vi "AddActions.vi"(0 "object in":refnum<class "StateReverse.lvclass">, 1 "StatesIn":T1[](array[typedef]), 5 "error in (no error)":errorcluster, 6 "StateStrings":string[](array[string]), 8 "StateActions":cluster{"StateActions":string[]}[](array[cluster]), 10 "StateComments":cluster{"StateActions":string[]}[](array[cluster])) -> (14 "object out":refnum<class "StateReverse.lvclass">, 15 "States":T1[](array[typedef]), 19 "error out":errorcluster)   [LabVIEW 2014, in "StateReverse.lvclass"]
uses:
  <resource>/Framework/Providers/Open_GDS/UML/StateReverse_class/StateReverse.lvclass
  <resource>/Framework/Providers/Open_GDS/UML/ReversedEngineering/ReversedEngineering StateMachineStateInfo.ctl
  <resource>/Framework/Providers/Open_GDS/UML/StateReverse_class/StateReverse.lvclass/StateReverse.ctl
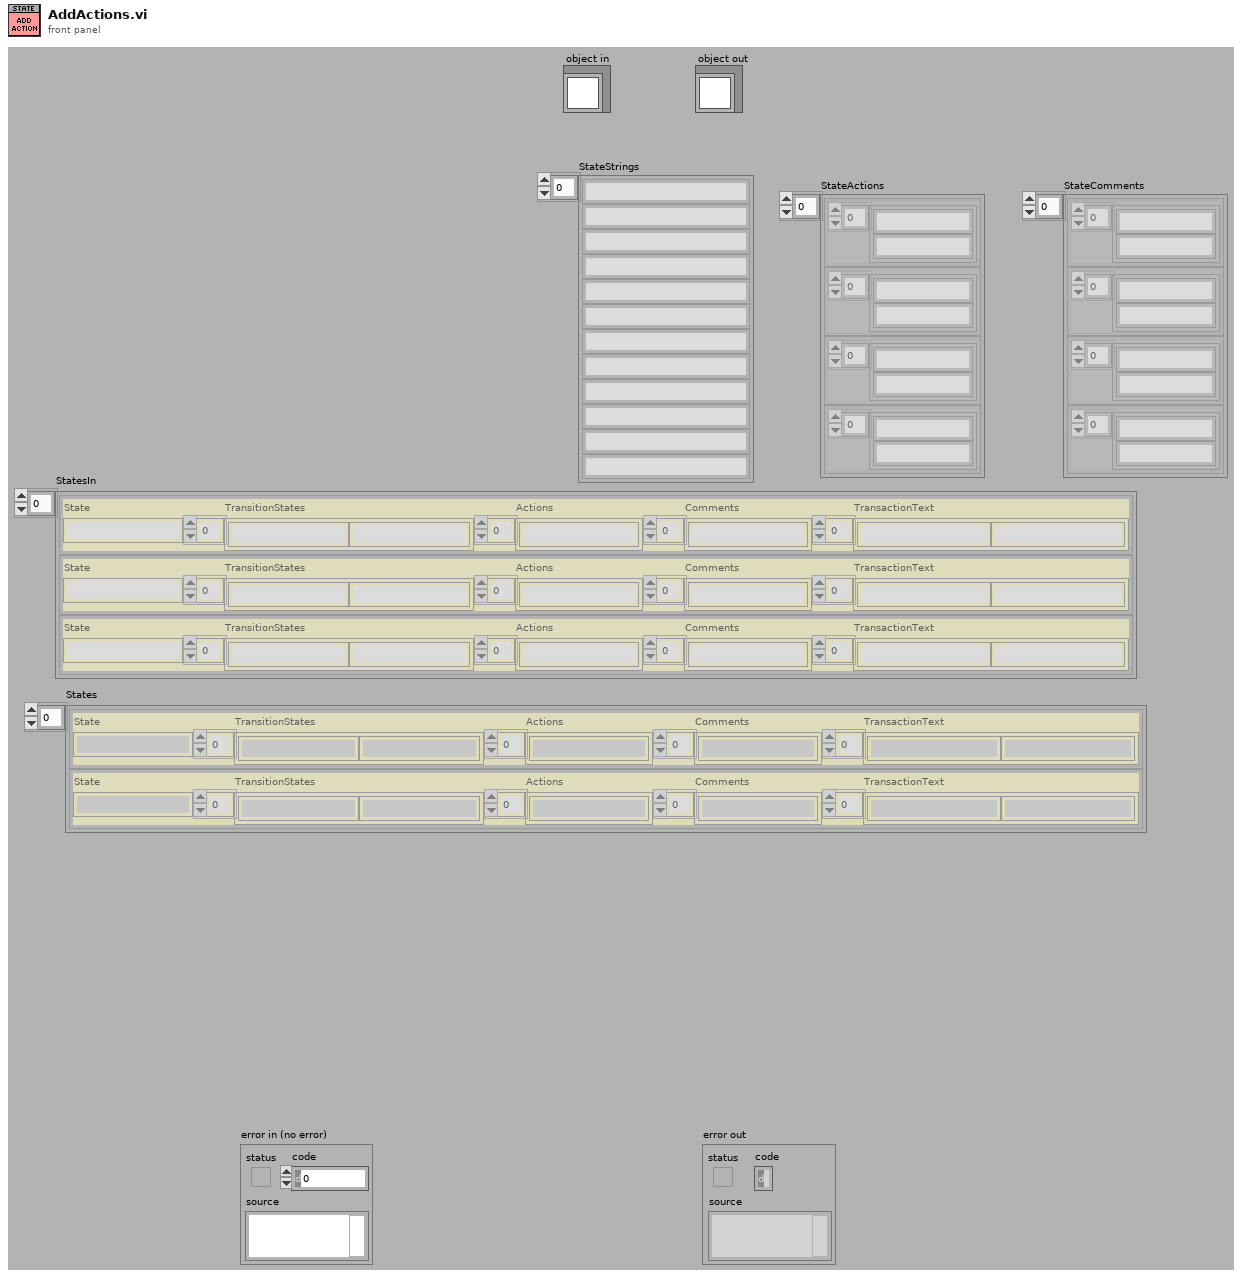
[diagram p1: front panel]
types:
  T1 = typedef "ReversedEngineering StateMachineStateInfo.ctl" = cluster{"State":string, "TransitionStates":string[], "Actions":string[], "Comments":string[], "TransactionText":string[]}
  T2 = typedef "StateReverse.lvclass/StateDetails.ctl" = cluster{"State":string, "NextStates":T3[], "QueueUsed":bool}
  T3 = typedef "StateReverse.lvclass/NextStateAction.ctl" = cluster{"State(s)":string, "StateAction":T4, "Arg(s)":string, "Comment(s)":string}
  T4 = typedef "StateReverse.lvclass/StateAction.ctl" = enum16{"Normal", "AddInBeggining", "AddInEnd", "AddIfNothingInQueue"}
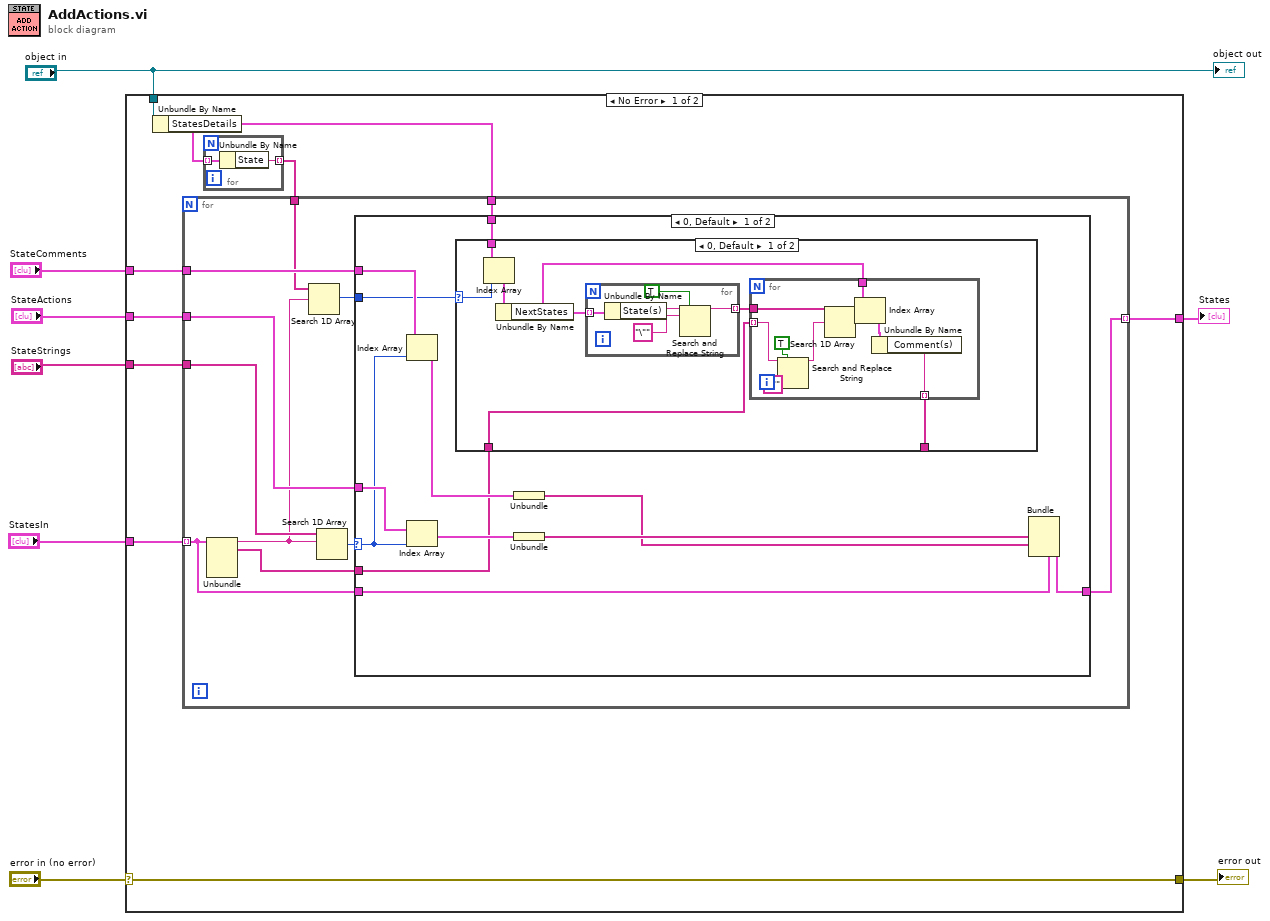
[diagram p0: block diagram]
diagram:
  n1 = case shown="No Error" "error in (no error)" {
    selector: "error in (no error)" -> [w14 w65]
    tunnel: [w14 w65] -> w7
    tunnel: "StatesIn" -> [w17 _]
    tunnel: [w15 _] -> w5
    tunnel: "StateStrings" -> [w16 _]
    tunnel: "StateActions" -> [w13 _]
    tunnel: "StateComments" -> [w12 _]
    tunnel: "object in" -> [w11 _]
    frame No Error {
      n2 = Unbundle By Name(w11) -> ("StatesDetails"=w9:T2[])
      n3 = for {
        tunnel: w9 -> [w19] mode=indexing
        tunnel: [w18] -> w10 mode=indexing
        n4 = Unbundle By Name(w19) -> ("State"=w18:string)
      }
      n5 = for {
        tunnel: w17 -> [w28] mode=indexing
        tunnel: w16 -> [w30]
        tunnel: [w21] -> w15 mode=indexing
        tunnel: w13 -> [w27]
        tunnel: w12 -> [w26]
        tunnel: w10 -> [w24]
        tunnel: w9 -> [w22]
        n6 = Unbundle(w28) -> ("State"=w25:string, "TransitionStates"=w20:string[])  [unwired: 3 out]
        n7 = Search 1D Array(1D array=w24, element=w25) -> (index of element=w23:i32)  [unwired: 1 in]
        n8 = Search 1D Array(1D array=w30, element=w25) -> (index of element=w29:i32)  [unwired: 1 in]
        n9 = case shown="0, Default" w29 {
          selector: w29 -> [w40 _]
          tunnel: w28 -> [w39 w64]
          tunnel: [w34 w64] -> w21
          tunnel: w27 -> [w42 _]
          tunnel: w26 -> [w41 _]
          tunnel: w23 -> [w33 _]
          tunnel: w22 -> [w32 _]
          tunnel: w20 -> [w31 _]
          frame 0, Default {
            n10 = Index Array(array=w41, index=w40) -> (element=w35:cluster{"StateActions":string[]})
            n11 = Index Array(array=w42, index=w40) -> (element=w38:cluster{"StateActions":string[]})
            n12 = case shown="0, Default" w33 {
              selector: w33 -> [w48 _]
              tunnel: w32 -> [w49 _]
              tunnel: w31 -> [w45 _]
              tunnel: [w43 _] -> _
              frame 0, Default {
                n13 = Index Array(array=w49, index=w48) -> (element=w47:T2)
                n14 = Unbundle By Name(w47) -> ("NextStates"=w44:T3[])
                n15 = for {
                  tunnel: w44 -> [w63] mode=indexing
                  tunnel: [w59] -> w46 mode=indexing
                  n16 = Unbundle By Name(w63) -> ("State(s)"=w62:string)
                  n17 = Search and Replace String(replace all?=TRUE ("replace all? (F)"), input string=w62, search string="\"") -> (result string=w59:string)  [unwired: 5 in, 3 out]
                }
                n18 = for {
                  tunnel: w46 -> [w58]
                  tunnel: w45 -> [w51] mode=indexing
                  tunnel: w44 -> [w56]
                  tunnel: [w54] -> w43 mode=indexing
                  n19 = Search and Replace String(replace all?=TRUE ("replace all? (F)"), input string=w51, search string="\"") -> (result string=w50:string)  [unwired: 5 in, 3 out]
                  n20 = Search 1D Array(1D array=w58, element=w50) -> (index of element=w57:i32)  [unwired: 1 in]
                  n21 = Index Array(array=w56, index=w57) -> (element=w55:T3)
                  n22 = Unbundle By Name(w55) -> ("Comment(s)"=w54:string)
                }
              }
              frame -1 {
              }
            }
            n23 = Unbundle(w35) -> ("StateActions"=w36:string[])
            n24 = Unbundle(w38) -> ("StateActions"=w37:string[])
            n25 = Bundle(cluster=w39, "Actions"=w37, "Comments"=w36) -> (w34:T1)  [unwired: 3 in]
          }
          frame -1 {
          }
        }
      }
    }
    frame Error {
    }
  }
  "error out" <- w7
  "States" <- w5
  "object out" <- "object in"
